vi "GetElement(Single).vi"(7 "Qualified Name":string, 8 "error in (no error)":errorcluster, 10 "Key":string, 11 "ConfigManager in":refnum<class "ConfigManager.lvclass">) -> (0 "error out":errorcluster, 1 "Value":string, 2 "Key":string, 3 "ConfigManager out":refnum<class "ConfigManager.lvclass">, 4 "found":bool)   [LabVIEW 2013, in "CfgManager.lvlib" / "ConfigManager.lvclass"]
uses:
  ConfigManager.lvclass
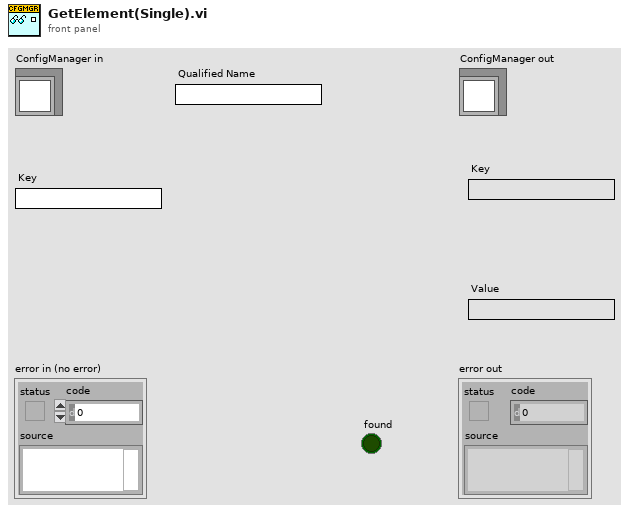
[diagram p1: front panel]
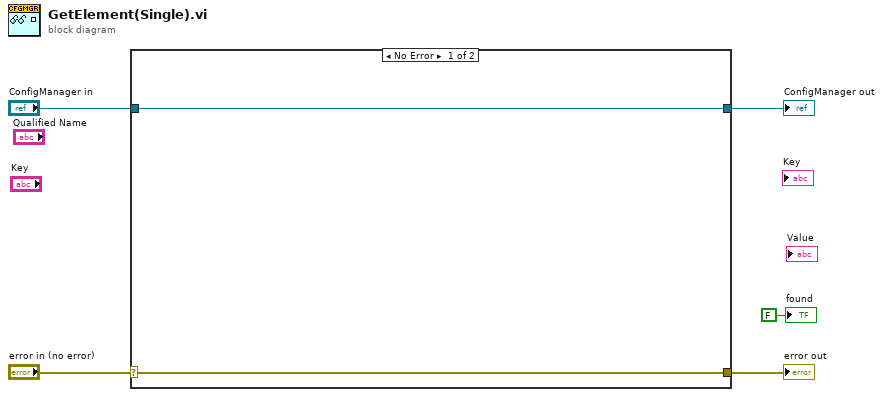
[diagram p0: block diagram]
diagram:
  n1 = case shown="No Error" "error in (no error)" {
    selector: "error in (no error)" -> [w6 w9]
    tunnel: [w6 w9] -> w4
    tunnel: [w7 w8] -> w2
    tunnel: "ConfigManager in" -> [w7 w8]
    frame No Error {
    }
    frame Error {
    }
  }
  "error out" <- w4
  "ConfigManager out" <- w2
  "found" <- FALSE ("found")
